vi "HandleMsg.vi"(7 "Rcv Msg Type":T1={"ID"=135, "Chksum"=123, "Unused"=0, "Length"=0, "Seq No"=0, "Msg Data"=[]}) -> (1 "ID":u8, 2 "Uint8 1":u8, 3 "Uint8 2":u8, 4 "Uint16 1":u16, 6 "Uint16 2":u16, 8 "Uint32":u32, 10 "Single 1":sgl format="%.2f", 13 "Double 2":dbl format="%.2f", 14 "Double 1":dbl format="%.2f", 15 "Single 2":sgl format="%.2f")   [LabVIEW 2016]
uses:
  RcvMsgType.ctl
  GlobalVars.vi
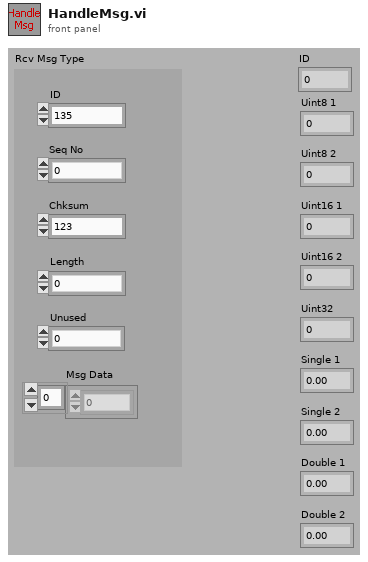
[diagram p1: front panel]
types:
  T1 = typedef "RcvMsgType.ctl" = cluster{"ID":u8, "Chksum":u16, "Unused":u16, "Length":u16, "Seq No":u8, "Msg Data":u8[]}
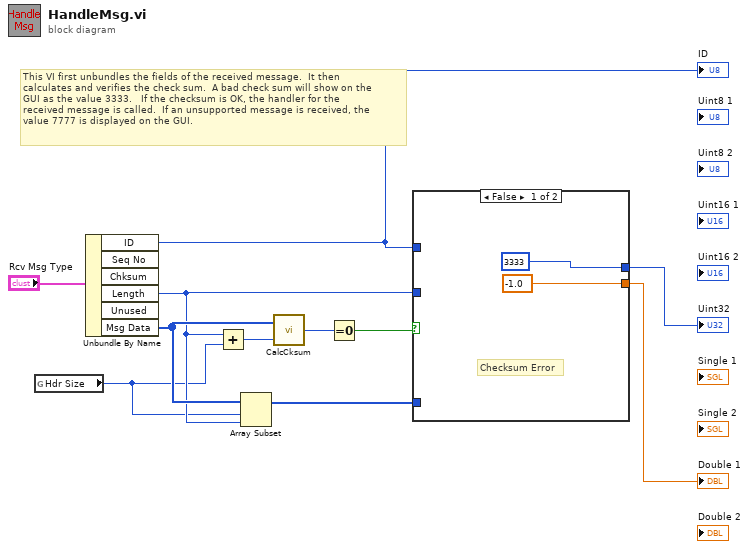
[diagram p0: block diagram]
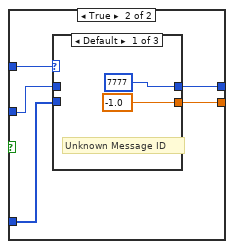
[diagram p2: hidden frame]
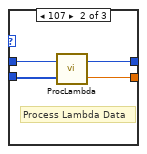
[diagram p3: hidden frame]
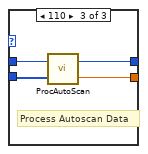
[diagram p4: hidden frame]
diagram:
  # "This VI first unbundles the fields of the received message.  It then\ncalculates and verifies the check sum.  A bad check sum will show on the\nGUI as the value 3333.   If the checksum is OK, the handler for the\nreceived message is called.  If an unsupported message is received, the\nvalue 7777 is displayed on the GUI."
  n1 = global read "GlobalVars.vi" "Hdr Size"() -> (w3:u8)
  n2 = Unbundle By Name "Unbundle By Name"("Rcv Msg Type") -> ("ID"=w5:u8, "Length"=w4:u16, "Msg Data"=w7:u8[])  [unwired: 3 out]
  "ID" <- w5
  n3 = Add(x=w4, y=w3) -> (x+y=w8:u16)
  n4 = Array Subset "Array Subset"(array=w7, index=w3, length=w4) -> (w6:u8[])
  n5 = call "CalcCksum.vi"("Byte Cnt"=w8, "Buffer"=w7) -> ("CkSum"=w10:u16)
  n6 = Equal To 0?(x=w10) -> (x = 0?=w9:bool)
  n7 = case shown="False" w9 {
    tunnel: w5 -> [_ w18]
    tunnel: w4 -> [_ w15]
    tunnel: w6 -> [_ w17]
    tunnel: [-1.0 w16] -> w2
    tunnel: [u32 3333 ("Lambda") w14] -> w1
    frame False {
      # "Checksum Error"
    }
    frame True {
      n8 = case shown="Default" w18 {
        tunnel: w17 -> [_ w23 w27]
        tunnel: [-1.0 ("Lambda") w22 w26] -> w16
        tunnel: w15 -> [_ w24 w28]
        tunnel: [u32 7777 ("Error") w21 w25] -> w14
        frame Default {
          # "Unknown Message ID"
        }
        frame 107 {
          # "Process Lambda Data"
          n9 = call "ProcLambda.vi"("Body"=w23, "Length"=w24) -> ("Lambda"=w22:dbl, "Error"=w21:u32)
        }
        frame 110 {
          # "Process Autoscan Data"
          n10 = call "ProcAutoScan.vi"("Body"=w27, "Length"=w28) -> ("AutoScan Data"=w26:dbl, "Error"=w25:u32)
        }
      }
    }
  }
  "Uint32" <- w1
  "Double 1" <- w2
